vi "Assemble Test Executive Builder ViewManager.vi"(5 "Active File Not Changed Tip Strip":string, 6 "Dirty Dot True":picture, 7 "Active File Changed Tip Strip":string, 9 "Active Path View":refnum<class "Test Executive Builder Active Path View.lvclass">, 10 "File Explorer View":refnum<class "File Explorer.lvclass">, 11 "Test Executive Builder View":refnum<class "Test Executive Builder View.lvclass">) -> (3 "Test Executive Builder ViewManager out":refnum<class "Test Executive Builder ViewManager.lvclass">)   [LabVIEW 2017, in "Test Executive Builder ViewManager.lvclass"]
uses:
  Test Executive Builder ViewManager.lvclass
  C:/Program Files/National Instruments/LabVIEW 2017/vi.lib/gpm_packages/@cs/mva-viewable/Source/IViewManager/IViewManager/IViewManager.lvclass
  Test Executive Builder View/Test Executive Builder View/Test Executive Builder View.lvclass
  C:/Program Files/National Instruments/LabVIEW 2017/vi.lib/gpm_packages/@cs/mva-viewable/Source/IViewable/IViewable/IViewable.lvclass
  <vilib>/gpm_packages/@cs/file-explorer-extension/Source/File Explorer/File Explorer/File Explorer.lvclass
  Active Path View/Test Executive Builder Active Path View/Test Executive Builder Active Path View.lvclass
  Dirty Dot View/Test Executive Builder Dirty Dot View/Test Executive Builder Dirty Dot View.lvclass
  Active Version View/Test Executive Builder Active Version View/Test Executive Builder Active Version View.lvclass
  Active Info View/Test Executive Builder Active Info View/Test Executive Builder Active Info View.lvclass
  <vilib>/gpm_packages/@cs/mva-viewable/Source/IViewManager/IViewManager Messages/Launch Nested Views Msg/Launch Nested Views Msg.lvclass/Launch Nested Views Msg.ctl
  <vilib>/gpm_packages/@cs/mva-viewable/Source/IViewManager/IViewManager/IViewManager.lvclass/IViewManager.ctl
  <vilib>/gpm_packages/@cs/mva-viewable/Source/IViewManager/IViewManager Messages/Launch Nested Views Msg/Pack Launch Nested Views Msg.vi
  <vilib>/gpm_packages/@cs/mva-viewable/Source/IViewManager/IViewManager Messages/Launch Nested Views Msg/Launch Nested Views Msg.lvclass
  <vilib>/gpm_packages/@cs/mva-viewable/Source/IViewManager/IViewManager/IViewManager.lvclass
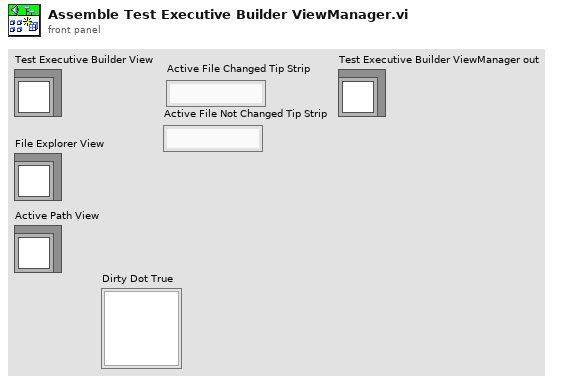
[diagram p1: front panel]
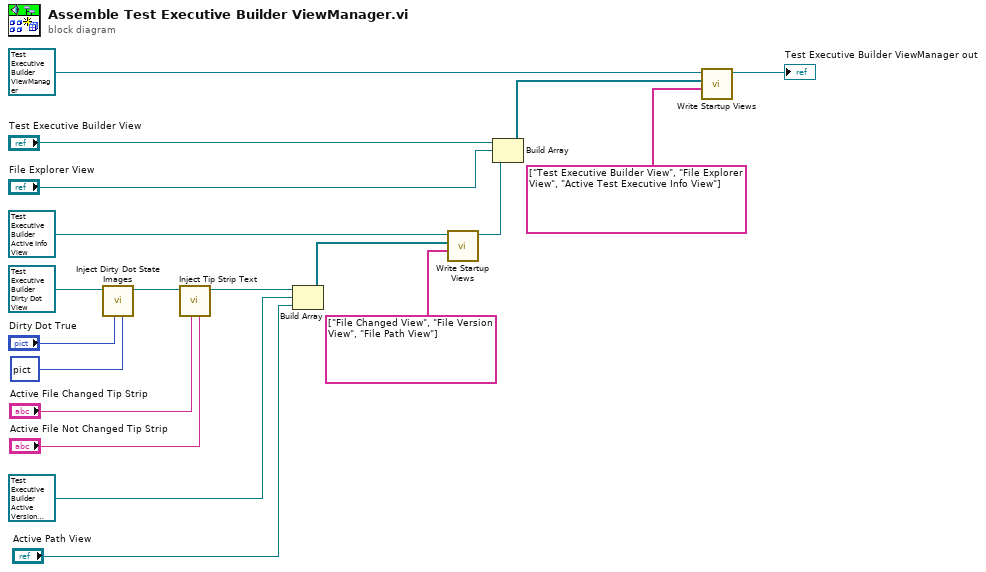
[diagram p0: block diagram]
diagram:
  n1 = call "Inject Dirty Dot State Images.vi"("Dirty Dot False"=picture data[5B], "Dirty Dot True"="Dirty Dot True", "Test Executive Builder Dirty Dot View in"=refnum<class "Test Executive Builder Dirty Dot View.lvclass"> refnum ("Test Executive Builder Dirty Dot View.lvclass")) -> ("Test Executive Builder Dirty Dot View out"=w4:refnum<class "Test Executive Builder Dirty Dot View.lvclass">)  [unwired: 8 in]
  n2 = call "Inject Tip Strip Text.vi"("Active File Not Changed Tip Strip"="Active File Not Changed Tip Strip", "Active File Changed Tip Strip"="Active File Changed Tip Strip", "Test Executive Builder Dirty Dot View in"=w4) -> ("Test Executive Builder Dirty Dot View out"=w3:refnum<class "Test Executive Builder Dirty Dot View.lvclass">)  [unwired: 8 in]
  n3 = Build Array(w3, refnum<class "Test Executive Builder Active Version View.lvclass"> refnum ("Test Executive Builder Active Version View.lvclass"), "Active Path View") -> (w10:refnum<class "IViewable.lvclass">[])
  n4 = call <vilib>:"Write Startup Views.vi"("View Labels"=string[] ["File Changed View", "File Version View", "File Path View"], "Startup Views"=w10, "IViewManager in"=refnum<class "Test Executive Builder Active Info View.lvclass"> refnum ("Test Executive Builder Active Info View")) -> ("IViewManager out"=w12:refnum<class "Test Executive Builder Active Info View.lvclass">)  [unwired: 8 in]
  n5 = Build Array("Test Executive Builder View", "File Explorer View", w12) -> (w15:refnum<class "IViewable.lvclass">[])
  n6 = call <vilib>:"Write Startup Views.vi"("View Labels"=string[] ["Test Executive Builder View", "File Explorer View", "Active Test Executive Info View"], "Startup Views"=w15, "IViewManager in"=refnum<class "Test Executive Builder ViewManager.lvclass"> refnum ("Test Executive Builder ViewManager out")) -> ("IViewManager out"=→"Test Executive Builder ViewManager out":refnum<class "Test Executive Builder ViewManager.lvclass">)  [unwired: 8 in]
